vi "Decimate (single shot, CDB).vi"(9 "averaging":bool, 10 "decimating factor":i32=1, 11 "X":cdb[](array[numeric])) -> (0 "error":i32, 3 "Decimated Array":cdb[](array[numeric]))   [LabVIEW 2014, in "NI_AALPro.lvlib"]
doc: "Decimates the input sequence <B>X</B> by the <B>decimating factor</B> and the <B>averaging</B> Boolean control. Wire data to the <B>X</B> input to determine the polymorphic instance to use or manually select the instance."
uses:
  NI_AALPro.lvlib
  lvanlys.dll
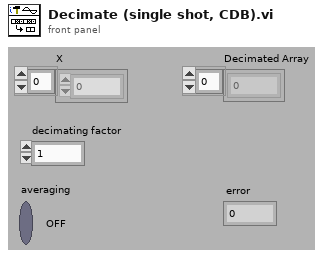
[diagram p1: front panel]
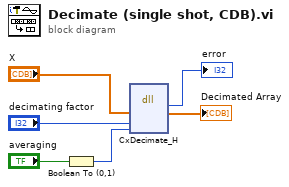
[diagram p0: block diagram]
diagram:
  n1 = Boolean To (0,1)(Boolean="averaging") -> (0, 1=w1:i16)
  n2 = dll-call lib="C:/Program Files (x86)/National Instruments/LabVIEW 2014/resource/lvanlys.*" fn="CxDecimate_H"("X"="X", "decimating factor"="decimating factor", "averaging"=w1) -> (→"error":i32, "X"=→"Decimated Array":cdb[])  [unwired: 5 in, 2 out]
